vi "Get Engine.vi"(8 "error in (no error)":errorcluster, 11 "Execution in":refnum<class "Execution.lvclass">) -> (0 "error out":errorcluster, 2 "Engine":T1, 3 "Execution out":refnum<class "Execution.lvclass">)   [LabVIEW 2020, in "TSS.lvlib" / "Execution.lvclass"]
uses:
  Execution.lvclass
  Engine/Typedefs/Session Handle.ctl
  Engine/Engine.lvclass
  Execution.lvclass/Execution.ctl
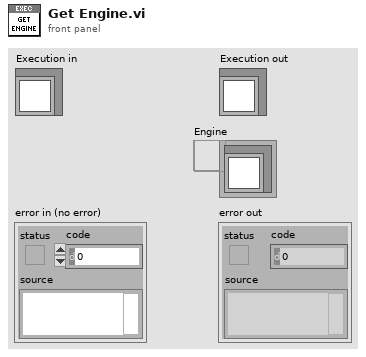
[diagram p1: front panel]
types:
  T1 = typedef "TSS.lvlib/Engine.lvclass/Session Handle.ctl" = refnum<data-value>
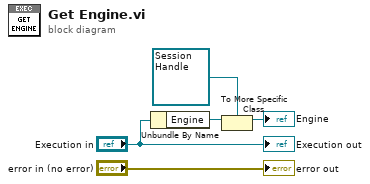
[diagram p0: block diagram]
diagram:
  n1 = Unbundle By Name("Execution in") -> ("Engine"=w3:refnum<data-value>)
  n2 = To More Specific Class(target class=T1 refnum ("Engine"), reference=w3) -> (specific class reference=→"Engine":T1)  [unwired: 1 in, 1 out]
  "error out" <- "error in (no error)"
  "Execution out" <- "Execution in"
